vi "Medidor_File_2.vi"() -> (0 "Tensão Fase B":dynamicdata(graph), 1 "Corrente Fase A":dynamicdata(graph), 2 "Tensão Fase A":dynamicdata(graph), 3 "Corrente Fase B":dynamicdata(graph), 4 "Tensão Fase c":dynamicdata(graph), 5 "Corrente Fase c":dynamicdata(graph), 6 "Timestamp":dynamicdata(graph))   [LabVIEW 2024]
panel:
  out "Fase C":string[][](table) caption="Table"
  out "Fase B":string[][](table) caption="Table"
  out "Fase A":string[][](table) caption="Table"
  out "Timestamp":string[][](table) caption="Table"
  out "All data":dynamicdata(graph)
  out "All data":string[][](table) caption="Table"
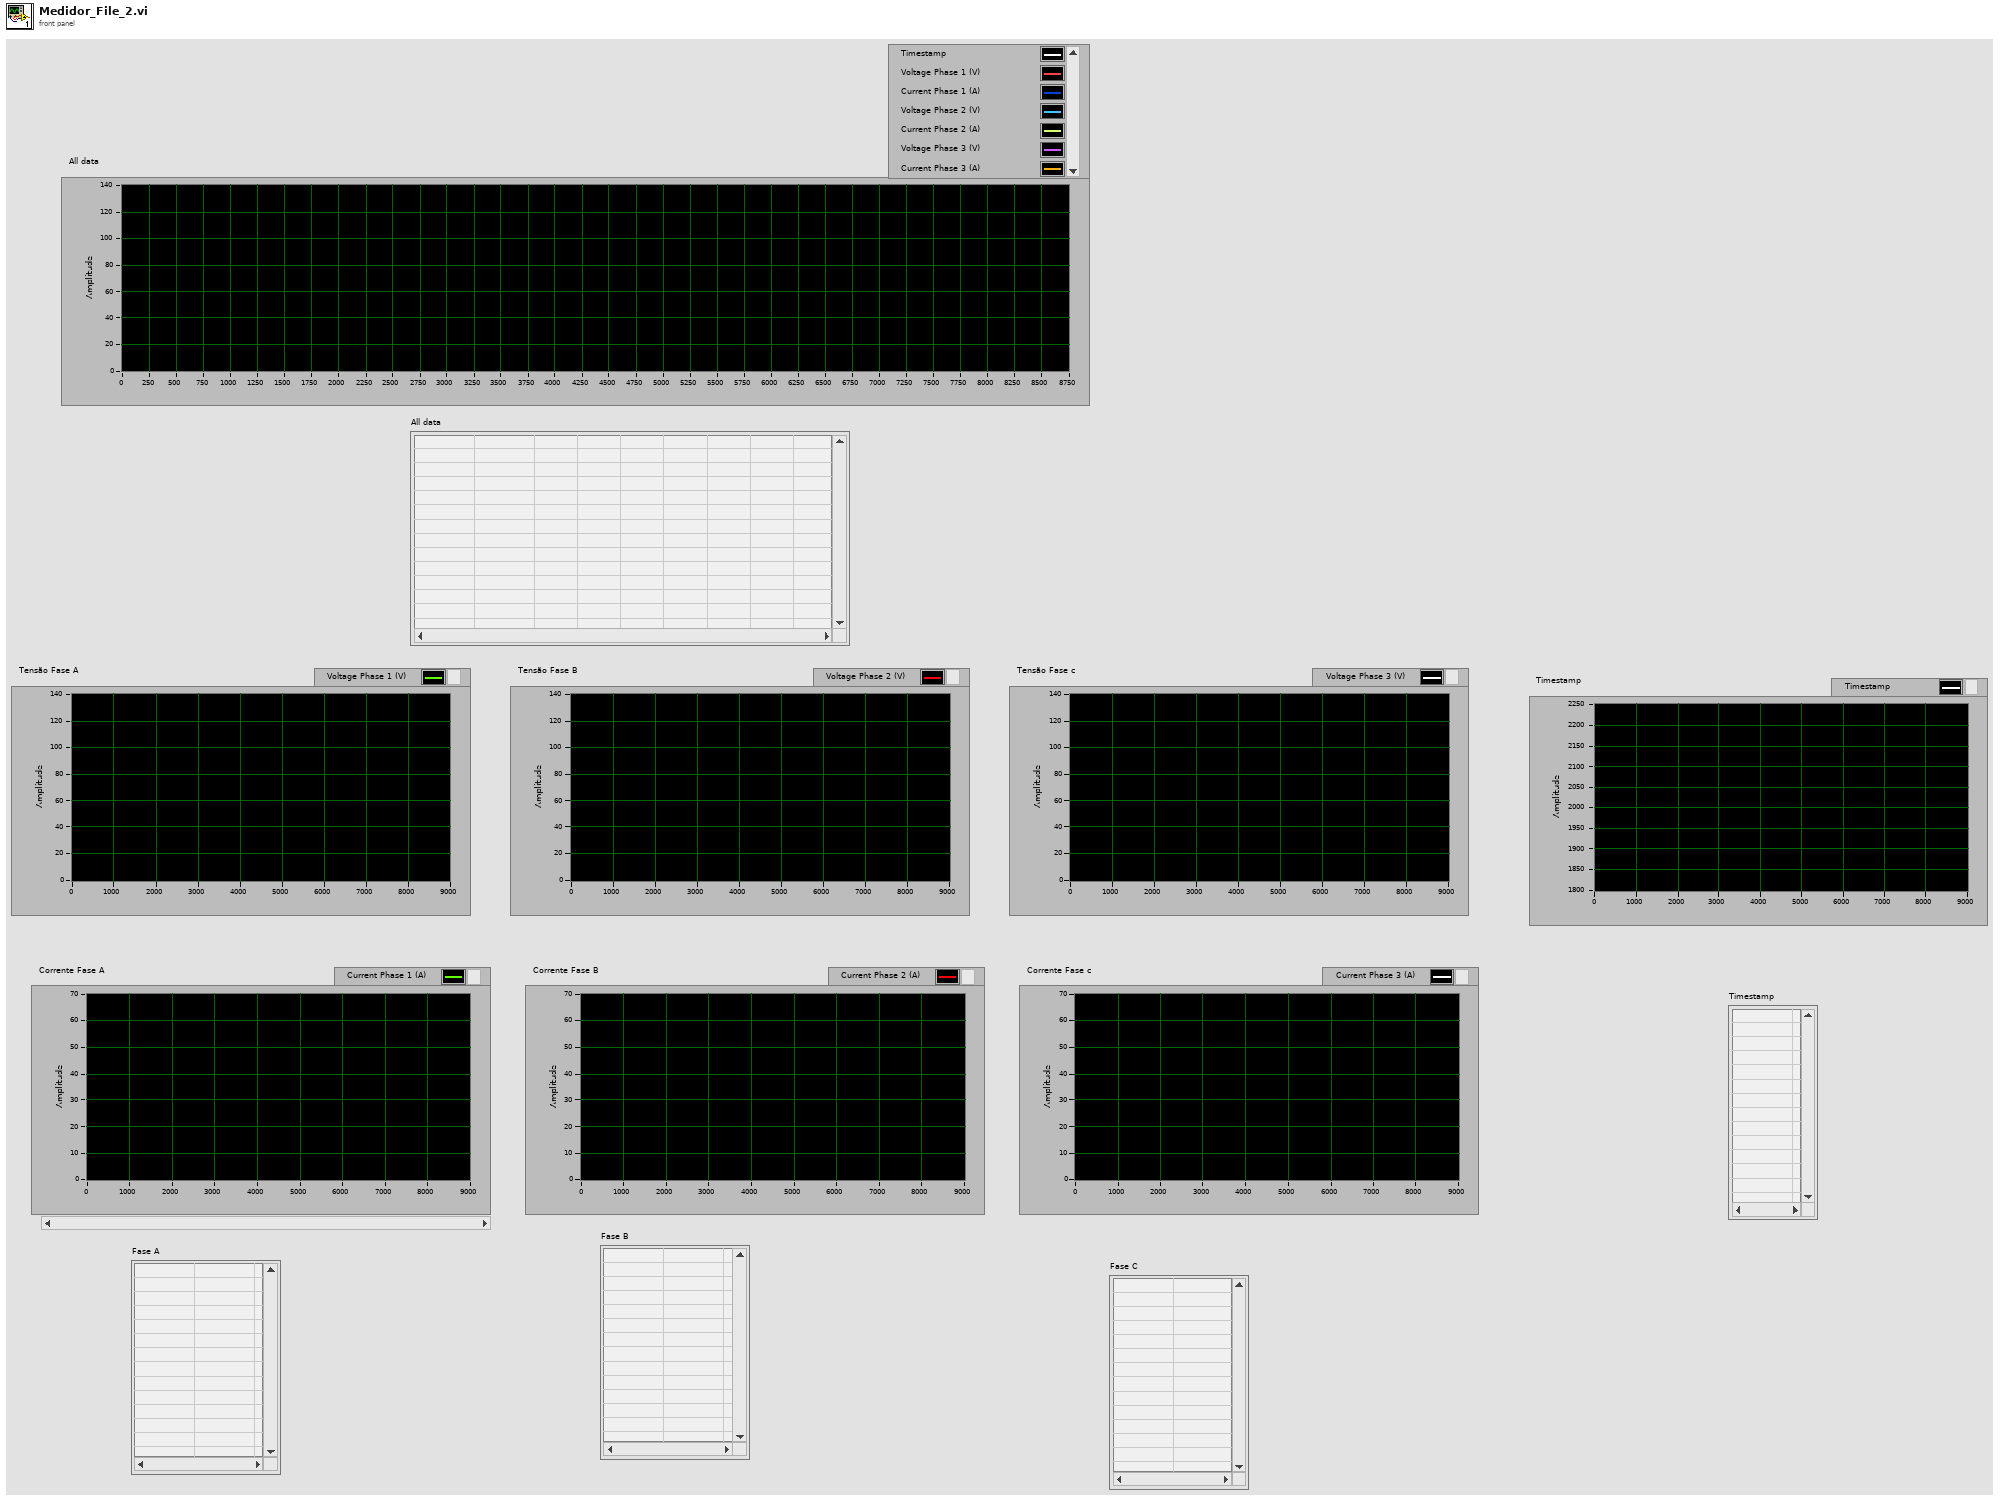
[diagram p1: front panel]
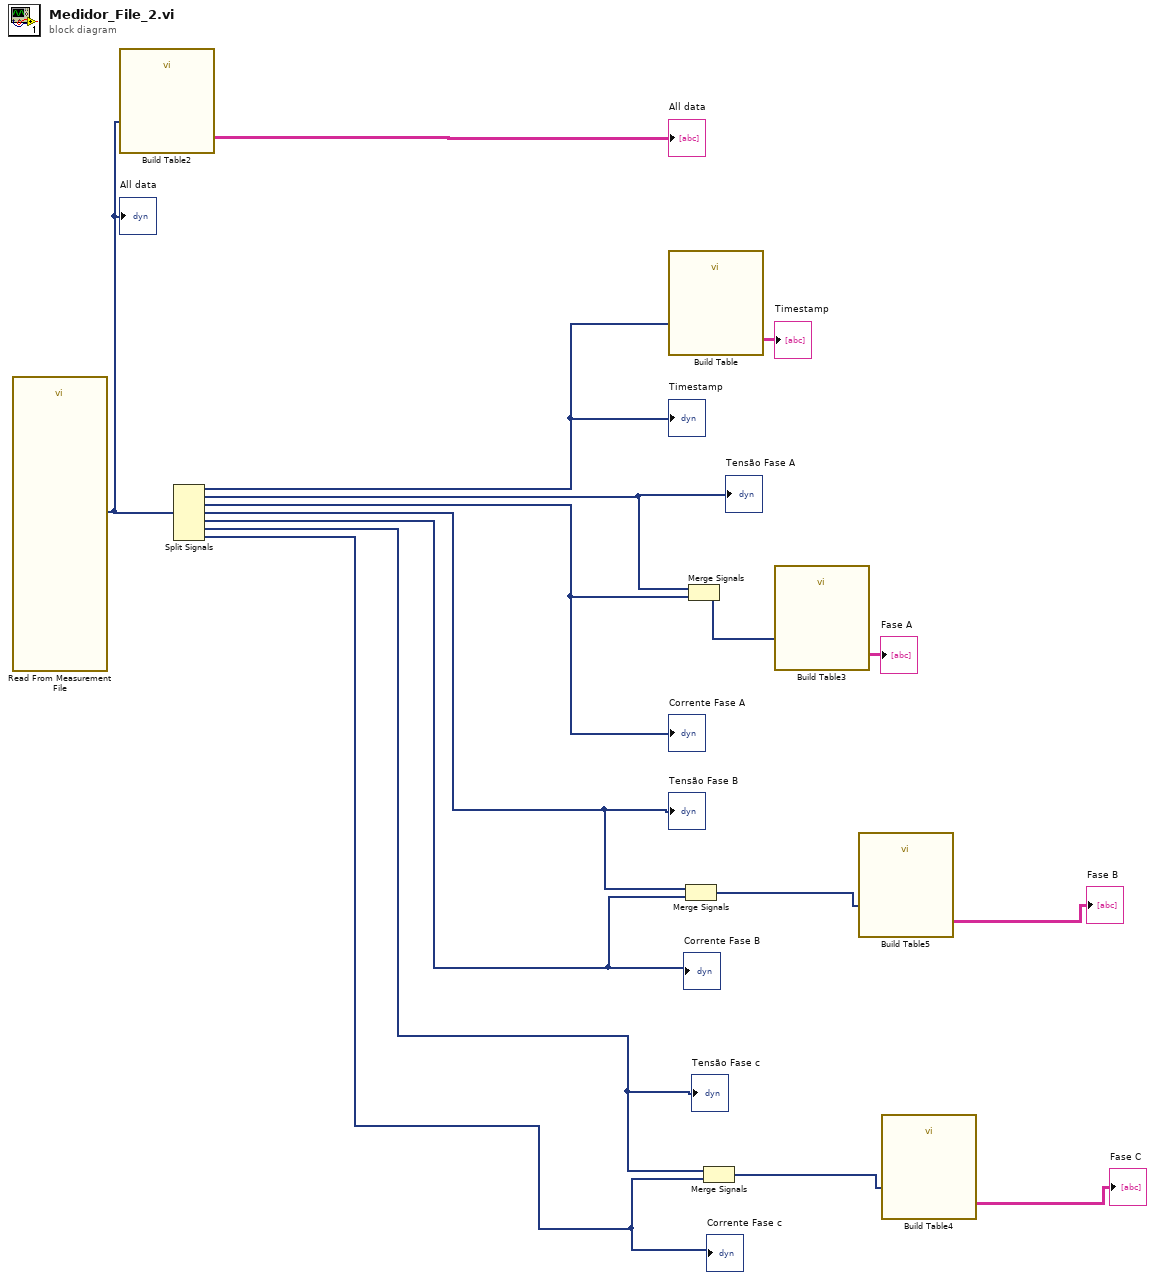
[diagram p0: block diagram]
diagram:
  n1 = call "Read From Measurement File"() -> ("Signals"=w15:dynamicdata)  [unwired: 6 in, 5 out]
  "All data" <- w15
  n2 = call "Build Table2"("Signals"=w15) -> ("Table"=→"All data":string[][])  [unwired: 4 in, 6 out]
  n3 = Split Signals(w15) -> (w13:dynamicdata, w4:dynamicdata, w3:dynamicdata, w11:dynamicdata, w10:dynamicdata, w6:dynamicdata, w5:dynamicdata)  [unwired: 7 in]
  "Timestamp" <- w13
  "Tensão Fase A" <- w4
  "Tensão Fase B" <- w11
  "Corrente Fase A" <- w3
  "Corrente Fase B" <- w10
  "Tensão Fase c" <- w6
  "Corrente Fase c" <- w5
  n4 = call "Build Table"("Signals"=w13) -> ("Table"=→"Timestamp":string[][])  [unwired: 4 in, 6 out]
  n5 = Merge Signals(w11, w10) -> (w2:dynamicdata)
  n6 = Merge Signals(w4, w3) -> (w1:dynamicdata)
  n7 = Merge Signals(w6, w5) -> (w8:dynamicdata)
  n8 = call "Build Table3"("Signals"=w1) -> ("Table"=→"Fase A":string[][])  [unwired: 4 in, 6 out]
  n9 = call "Build Table5"("Signals"=w2) -> ("Table"=→"Fase B":string[][])  [unwired: 4 in, 6 out]
  n10 = call "Build Table4"("Signals"=w8) -> ("Table"=→"Fase C":string[][])  [unwired: 4 in, 6 out]
